vi "Crear DAQ Task.vi"(8 "error in (no error)":errorcluster, 11 "DAQ DI in":refnum<class "DAQ DI.lvclass">) -> (0 "error out":errorcluster, 3 "DAQ DI out":refnum<class "DAQ DI.lvclass">)   [LabVIEW 2020, in "DAQ DI.lvlib" / "DAQ DI.lvclass"]
uses:
  DAQ DI.lvclass
  DAQ DI.lvclass/DAQ DI.ctl
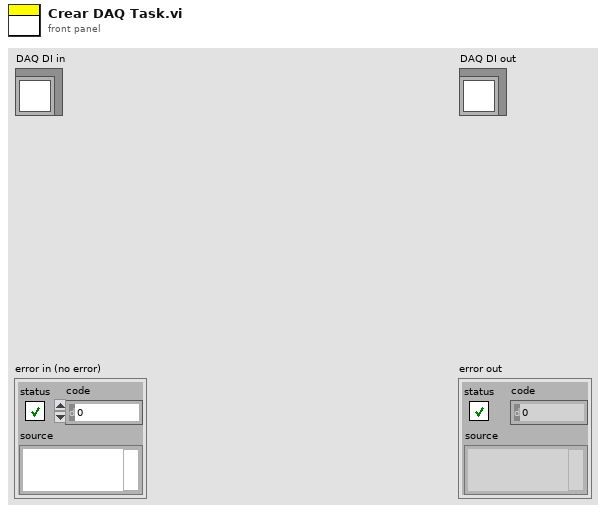
[diagram p1: front panel]
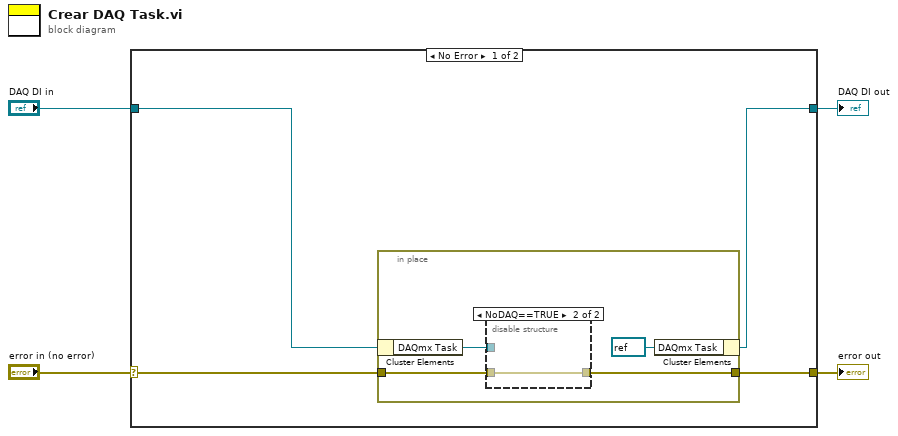
[diagram p0: block diagram]
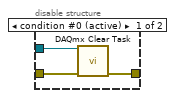
[diagram p2: hidden frame]
diagram:
  n1 = case shown="No Error" "error in (no error)" {
    selector: "error in (no error)" -> [w8 w18]
    tunnel: [w7 w18] -> w3
    tunnel: [w5 w17] -> w1
    tunnel: "DAQ DI in" -> [w6 w17]
    frame No Error {
      n2 = in-place {
        in-place-border: w8 -> [w12]
        in-place-border: [w11] -> w7
        n3 = in-place-cluster #1(w6) -> ("DAQmx Task"=w10:refnum<k21>)
        n4 = disable-structure shown="NoDAQ==TRUE" {
          disable-tunnel: w12 -> [w15 w16]
          disable-tunnel: [w14 w16] -> w11
          disable-tunnel: w10 -> [w13 _]
          frame condition #0 (active) {
            n5 = call <vilib>:"DAQmx Clear Task.vi"("task in"=w13, "error in"=w15) -> ("error out"=w14:errorcluster)  [unwired: 13 in]
          }
          frame condition #1 {
          }
        }
        n6 = in-place-cluster #1("DAQmx Task"=refnum<k21> refnum) -> (w5:refnum<class "DAQ DI.lvclass">)
      }
    }
    frame Error {
    }
  }
  "error out" <- w3
  "DAQ DI out" <- w1
